vi "test123.vi"() -> ()   [LabVIEW 2016]
uses:
  <vilib>/DAQmx/write.llb/DAQmx Write (Digital Bool 1Line 1Point).vi
  <vilib>/DAQmx/create/channels.llb/DAQmx Create Channel (DO-Digital Output).vi
  <vilib>/DAQmx/miscellaneous.llb/DAQmx Fill In Error Info.vi
  <vilib>/DAQmx/create/channels.llb/DAQmx Create Channel (DI-Digital Input).vi
panel:
  in  "stop":bool
  out "?":bool
  in  "Out":bool
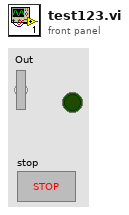
[diagram p1: front panel]
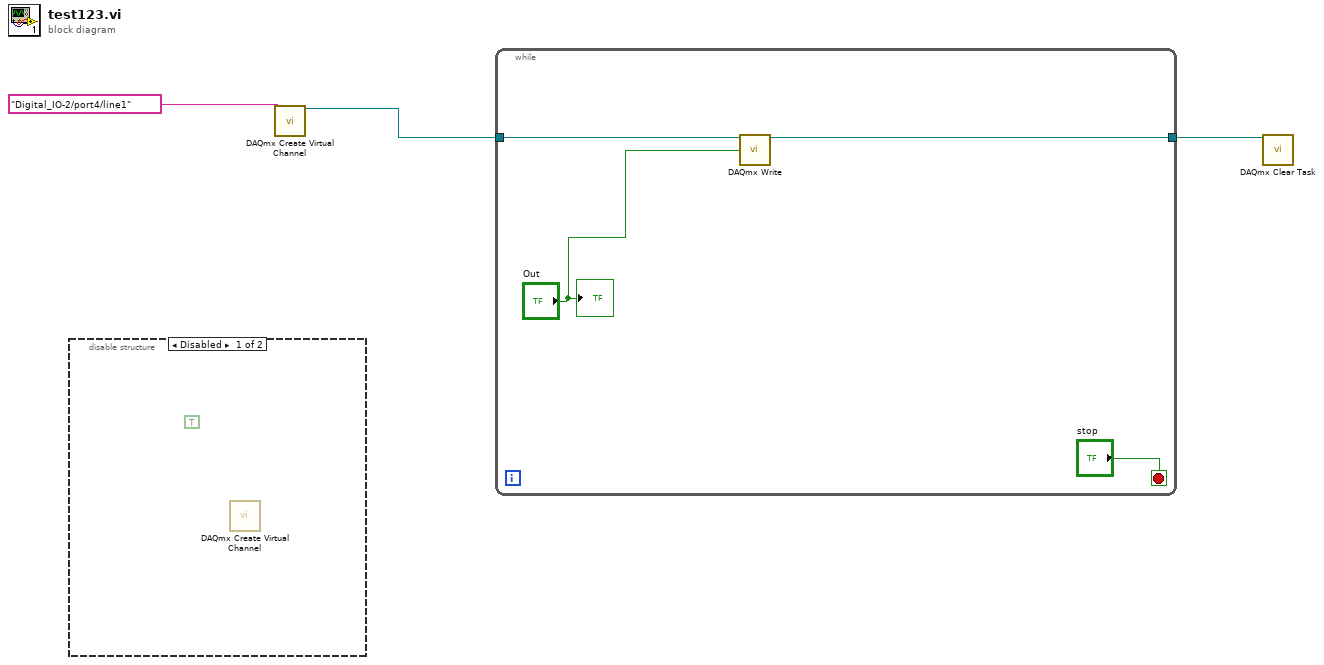
[diagram p0: block diagram]
diagram:
  n1 = disable-structure shown="Disabled" {
    frame Disabled {
      (unwired) TRUE ("data")
      n2 = call-poly <vilib>:"DAQmx Create Virtual Channel.vi"() -> ()  [unwired: 14 in, 2 out]
    }
    frame Enabled {
    }
  }
  n3 = call-poly <vilib>:"DAQmx Create Virtual Channel.vi"("lines"=tag "Digital_IO-2/port4/line1") -> ("task out"=w1:refnum<k21>)  [unwired: 13 in, 1 out]
  n4 = while {
    tunnel: [w7] -> w3
    tunnel: w1 -> [w5]
    stop <- "stop" stop-if-true
    n5 = call-poly <vilib>:"DAQmx Write.vi"("task/channels in"=w5, "data"="Out") -> ("task out"=w7:refnum<k21>)  [unwired: 11 in, 2 out]
    "?" <- "Out"
  }
  n6 = call <vilib>:"DAQmx Clear Task.vi"("task in"=w3) -> ()  [unwired: 14 in, 1 out]
